vi "seebeck.vi"() -> ()   [LabVIEW 2023]
uses:
  <instrlib>/Keithley 622x LV 2009/Keithley 622x.lvlib
  <instrlib>/Keithley 622x LV 2009/Utility/Typedefs/KE622x -- Instrument Type.ctl
  <vilib>/Analysis/NI_AALBase.lvlib
  <vilib>/Analysis/1siggen.llb/Ramp Pattern by Samples.vi
  Global Variables/MQM Data Transfer All.vi
  <vilib>/Analysis/baseanly.llb/Mean (DBL).vi
  Typedefs/Kxx_Kxy_state_machine_cases.ctl
  Global Variables/Thermometers.vi
  <vilib>/Utility/file.llb/Read Delimited Spreadsheet (DBL).vi
  <vilib>/Instr/_visa.llb/VISA Configure Serial Port (Instr).vi
  <vilib>/Utility/file.llb/Write To Spreadsheet File (string).vi
  Global Variables/KE2182 Voltage.vi
panel:
  in  "Seebeck Voltage Array":dbl[](array[numeric])
  in  "Seebeck coeff data":dbl[](array[numeric])
  in  "T_avg data":dbl[](array[numeric])
  in  "dTxx":dbl
  in  "HTR Power":dbl
  in  "T_avg":dbl
  in  "T_H Array":dbl[](array[numeric])
  in  "T_C Array":dbl[](array[numeric])
  in  "Seebeck Voltage":dbl
  in  "?":enum32{"Setup", "Plotting", "Error Readouts"}(tab)
  in  "DeltaT (fraction of tsp)":dbl=0.05
  in  "Heater Current File (H, T, current)":path
  out "Heater Current \nArray":dbl[](array[numeric])
  out "Ramp Pattern":dbl[](array[numeric])
  in  "Tstart (K)":dbl=3.0
  in  "Tend (K)":dbl=4.0
  in  "Steps":i16=2
  in  "Log (on)\nLin (off) (Temperature setpoints)":bool=TRUE
  in  "Initial Heater Current (A)":dbl=1e-06
  in  "Hstart (Oe)":dbl
  in  "Hend (Oe)":dbl
  in  "Field Steps":i16=1
  in  "Log (on)\nLin (off)  (Field setpoints)":bool
  in  "Test?":bool
  in  "Calibration Only?":bool
  in  "Exchange gas?":bool
  in  "Preset Heater Current Array?":bool
  in  "T Current Source":refnum<visa-resource-name>="6221B"
  in  "HTR Current Source":refnum<visa-resource-name>="CS580-1"
  in  "Thermometer Frequency (Hz)":string="37"
  in  "Initial Thermometer Current (A)":string="1.4142e-7"
  in  "Final Field (Oe)":dbl
  in  "Final Temperature (K)":dbl=1.7
  in  "Filename":path=path "C:/User Data/Luke/Kxx/NaYSe2/NaYSe2_1p7_100K_log_100_9T_8_23_21"
  in  "Heater Only?":bool
  in  "Running avg size":dbl=500.0 format="%#_13g"
  in  "std/mean thresh":dbl=1e-05 format="%#_13g"
  in  "slope/mean thresh":dbl=1e-07 format="%#_13g"
  out "Seebeck Coeff Plot":cluster{dbl[], dbl[]}(graph)
  out "All Data":cluster{dbl[], dbl[]}[](graph)
  in  "Finish":bool
  out "Data Rate (ms)":u32
  in  "Delay (ms)":dbl=300.0
  in  "Quick Data Recording":bool=TRUE
  out "Tsp":dbl
  out "HTR_Current":dbl
  out "Mask":dbl
  out "Seebeck Voltage":dbl
  out "T_H":dbl
  out "T_C1":dbl
  out "I_therm":dbl
  out "T_C2":dbl
  in  "Display Elements":cluster{"X":bool, "Y":bool, "Name":u16}[](array[cluster]) {"Name" items=["Time (ms)", "Temperature (K)", "Field (T)", "LI_1_X", "LI_1_theta", "LI_2_X", "LI_2_theta", "LI_3_X", "LI_3_theta", "DC_V", "DC_I", "mask", "tsp", "I_therm", "T_H", "T_C1", "T_C2", "Fieldsp"]}
  in  "X-Axis":u16(ring) items=["Linear", "Reciprocal", "Log10"]
  in  "Y-Axis":u16(ring) items=["Linear", "Reciprocal", "Log10"]
  out "Fieldsp":dbl
  out "Global Stop":bool
  out "Thermometers":cluster{"T_H":dbl, "T_C1":dbl, "T_C2":dbl}
  out "QD error out":errorcluster
  out "KE6221 error out":errorcluster
  # "TURN ON HIGH VACUUM!"
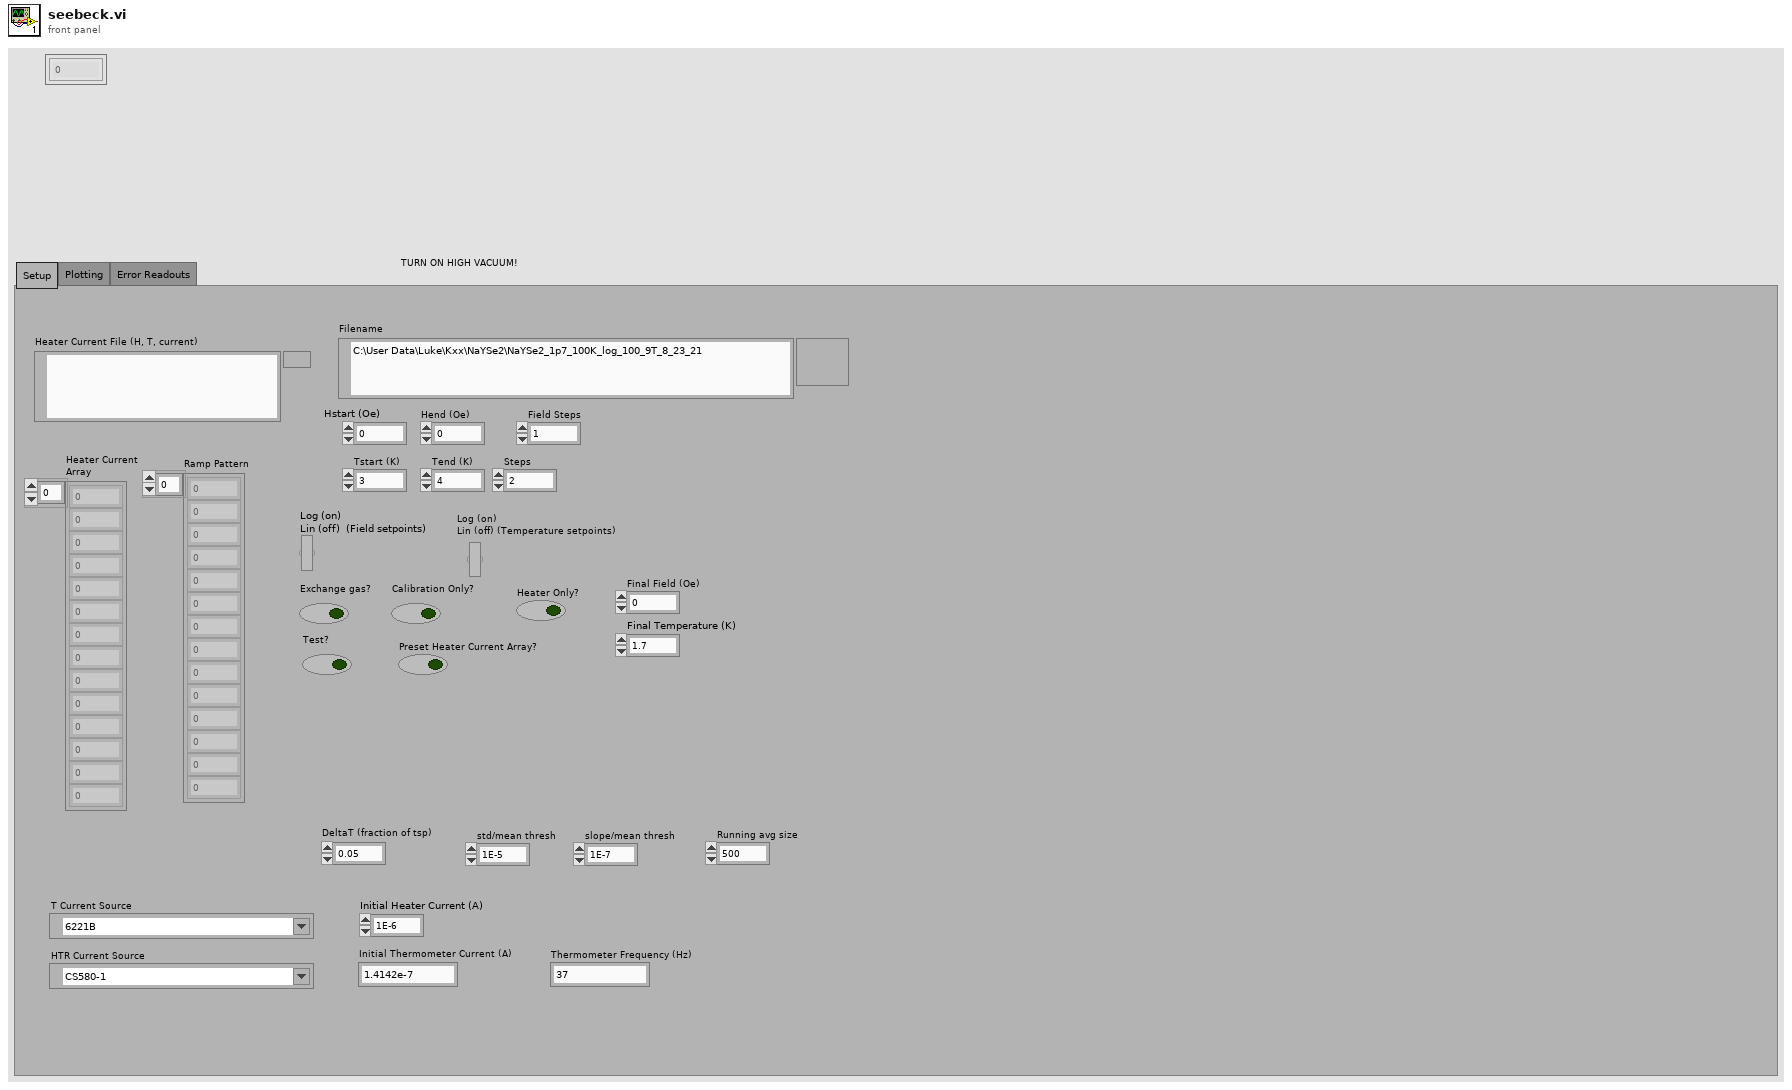
[diagram p1: front panel]
types:
  T1 = typedef "Keithley 622x.lvlib/KE622x -- Instrument Type.ctl" = enum16{"KE6220", "KE6221"}
  T2 = typedef "Kxx_Kxy_state_machine_cases.ctl" = enum16{"Initialize", "Wait to Stabilize (no heat)", "Measure (no heat)", "Turn on Heater, stabilize", "Measure (heat)", "Turn off Heater", "Assign Heater Current", "Plot", "End"}
  T3 = cluster{"T_avg data":dbl[], "Seebeck coeff data":dbl[]}
  T4 = cluster{"T_avg":dbl, "dTxx":dbl, "HTR Power":dbl, "Seebeck Voltage":dbl, "T_H Array":dbl[], "T_C Array":dbl[], "Seebeck Voltage Array":dbl[], "error out":errorcluster}
  T5 = typedef "ZI_Frontpanel_All.ctl" = cluster{"Lockin 1 Demod 0":cluster{"R(V)":dbl, "Theta (deg)":dbl, "Timestamp (ms)":u32, "X(V)":dbl, "Y(V)":dbl, "frequency (Hz)":dbl, "output voltage (V)":dbl}, "Lockin 2 Demod 0":cluster{"R(V)":dbl, "Theta (deg)":dbl, "Timestamp (ms)":u32, "X(V)":dbl, "Y(V)":dbl, "frequency (Hz)":dbl, "output voltage (V)":dbl}, "Lockin 3 Demod 0":cluster{"R(V)":dbl, "Theta (deg)":dbl, "Timestamp (ms)":u32, "X(V)":dbl, "Y(V)":dbl, "frequency (Hz)":dbl, "output voltage (V)":dbl}, "Lockin 4 Demod 0":cluster{"R(V)":dbl, "Theta (deg)":dbl, "Timestamp (ms)":u32, "X(V)":dbl, "Y(V)":dbl, "frequency (Hz)":dbl, "output voltage (V)":dbl}, "LI1 active":bool, "LI2 active":bool, "LI3 active":bool, "LI4 active":bool}
  T6 = typedef "PPMS_Status.ctl" = cluster{"Field":cluster{"Field (T)":dbl, "Field stable":bool, "Timestamp (ms)":u32}, "Temperature":cluster{"Temperature (K)":dbl, "Temperature stable":bool, "Timestamp (ms)":u32}}
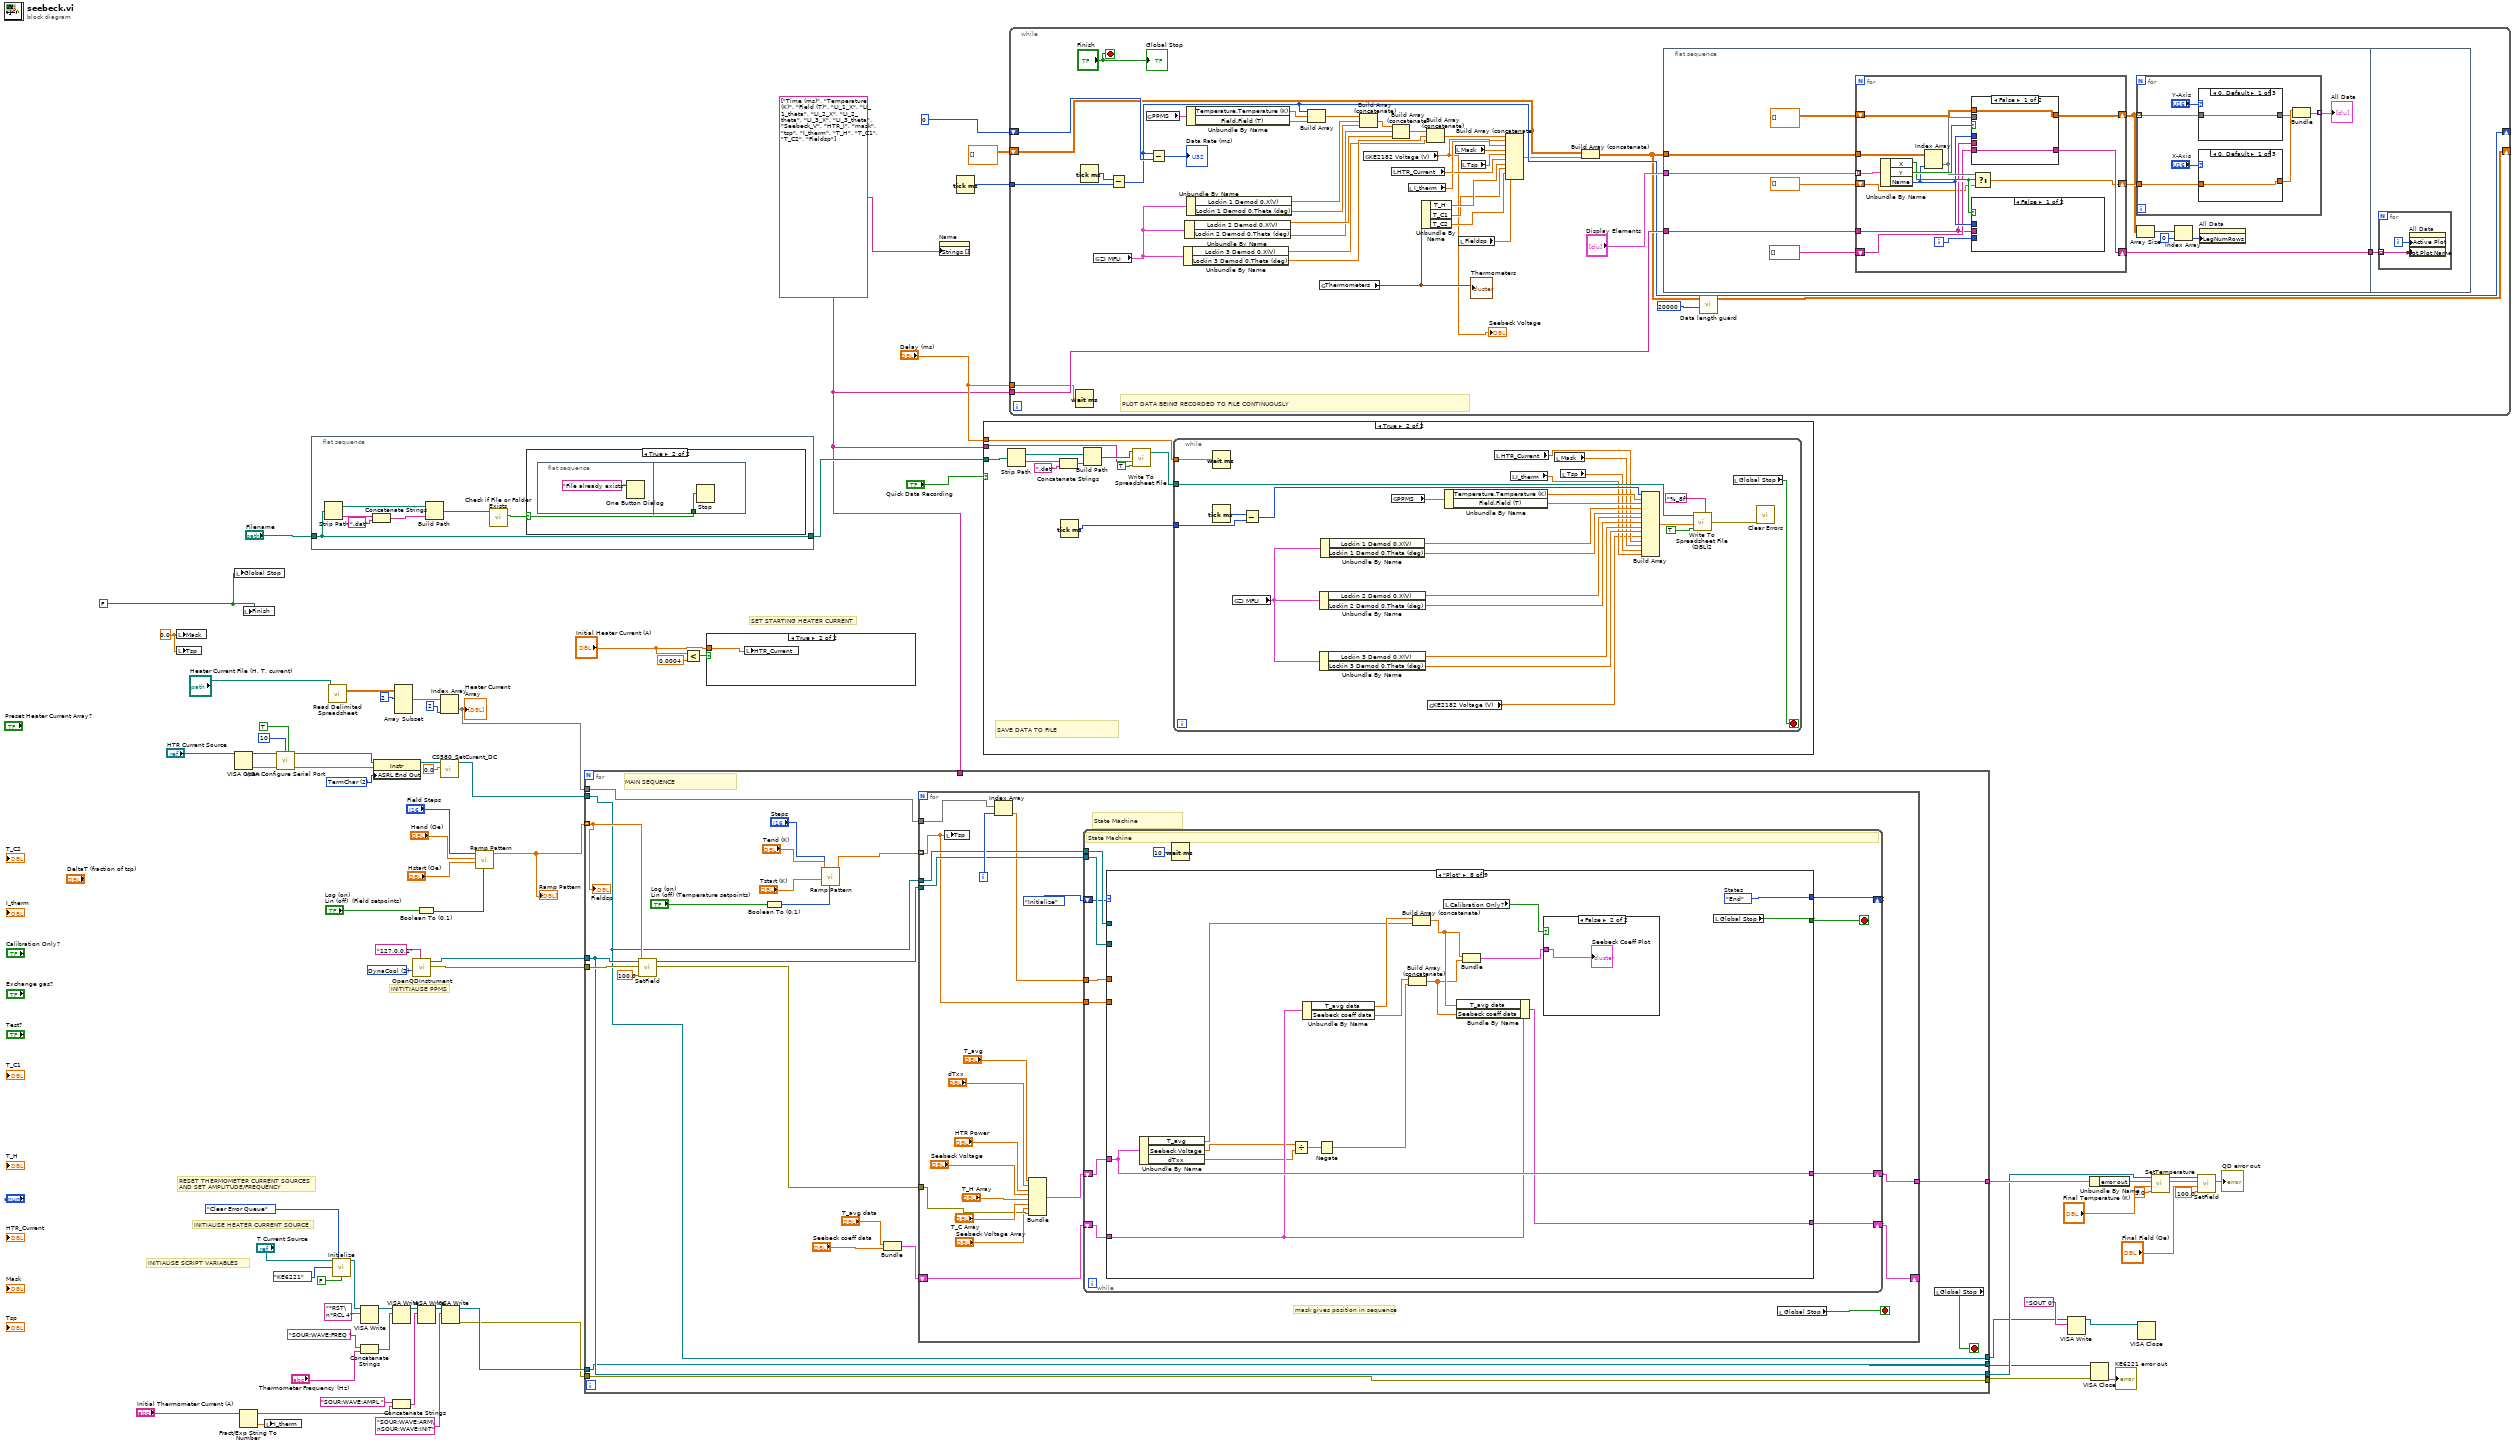
[diagram p0: block diagram]
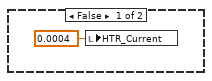
[diagram p2: hidden frame]
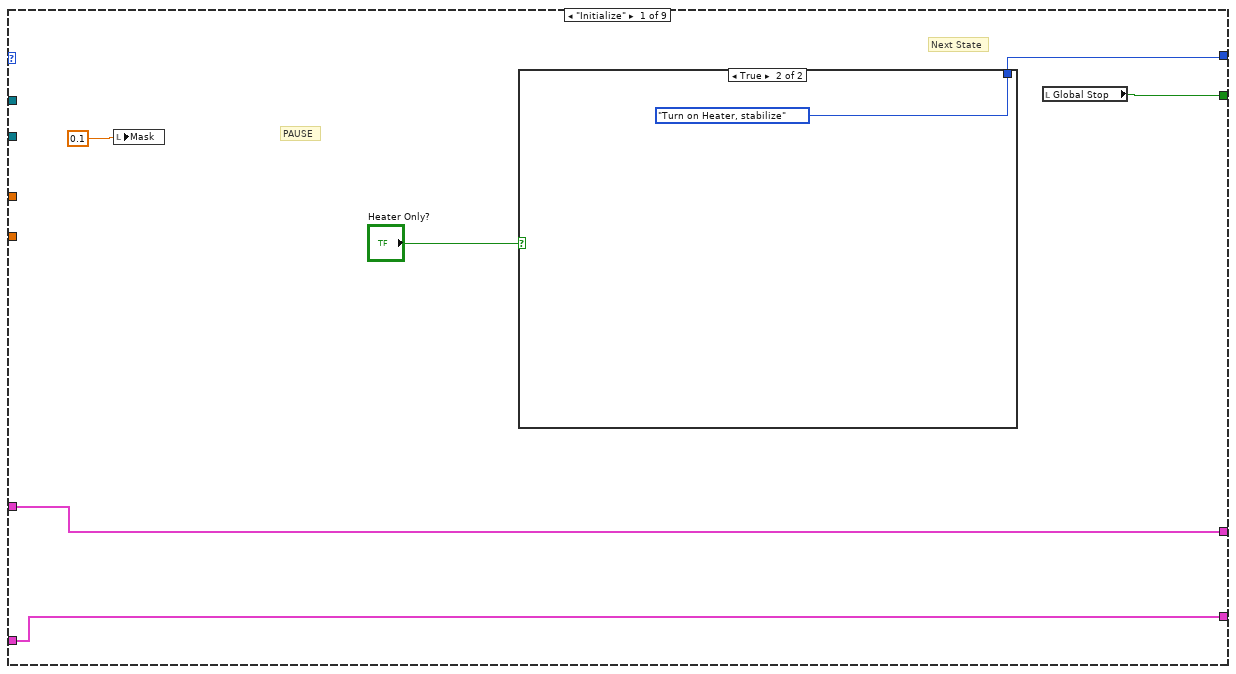
[diagram p4: hidden frame]
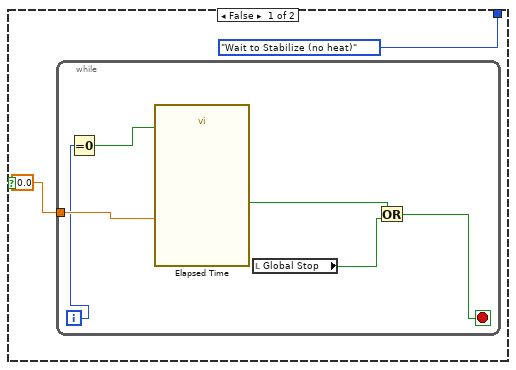
[diagram p5: hidden frame]
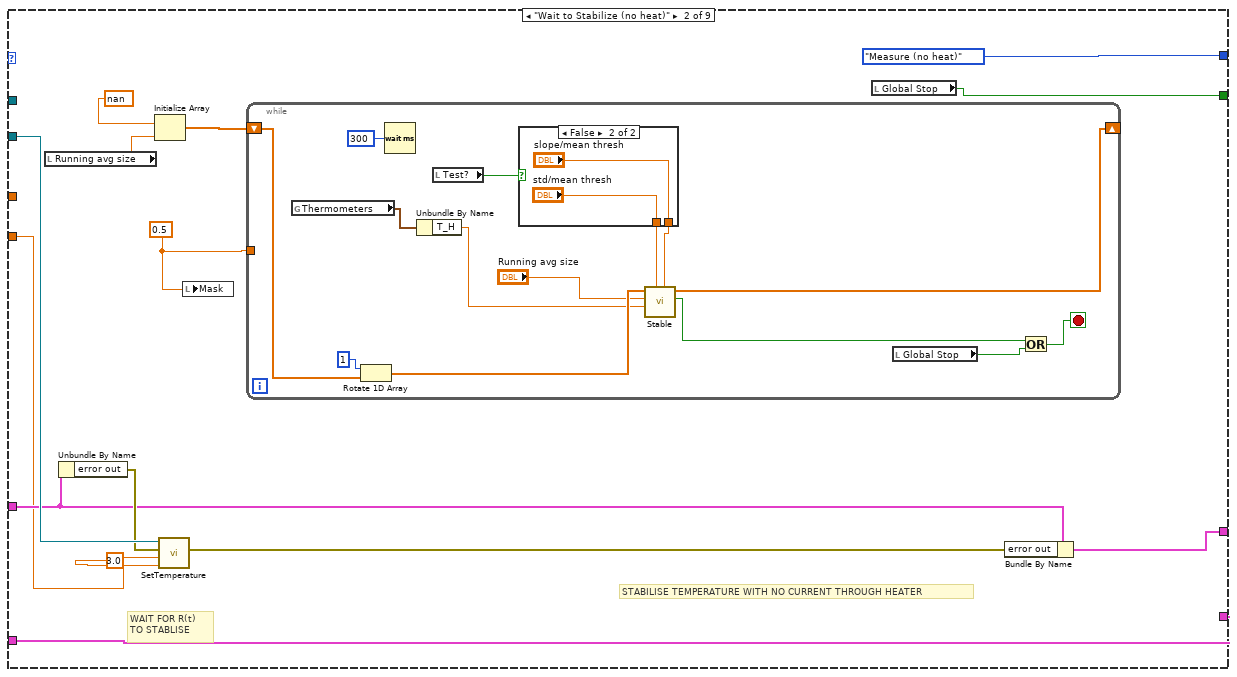
[diagram p6: hidden frame]
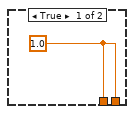
[diagram p7: hidden frame]
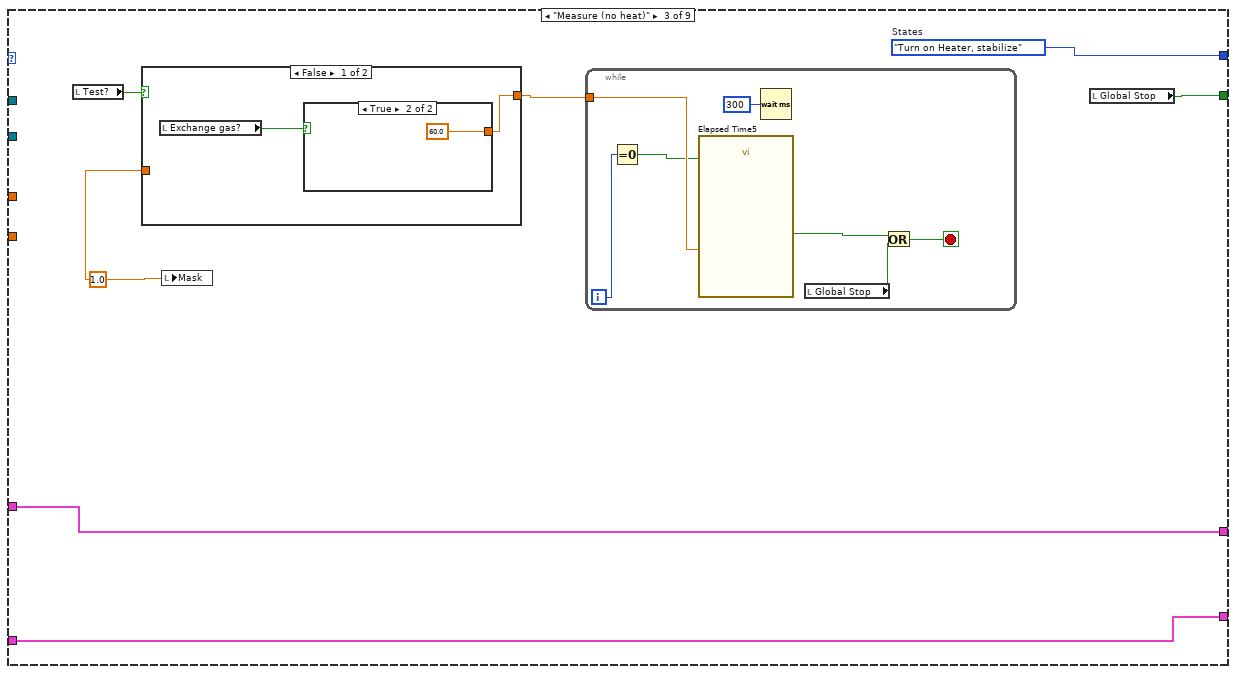
[diagram p8: hidden frame]
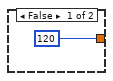
[diagram p9: hidden frame]
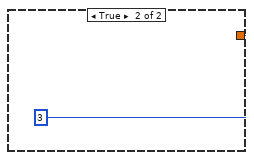
[diagram p10: hidden frame]
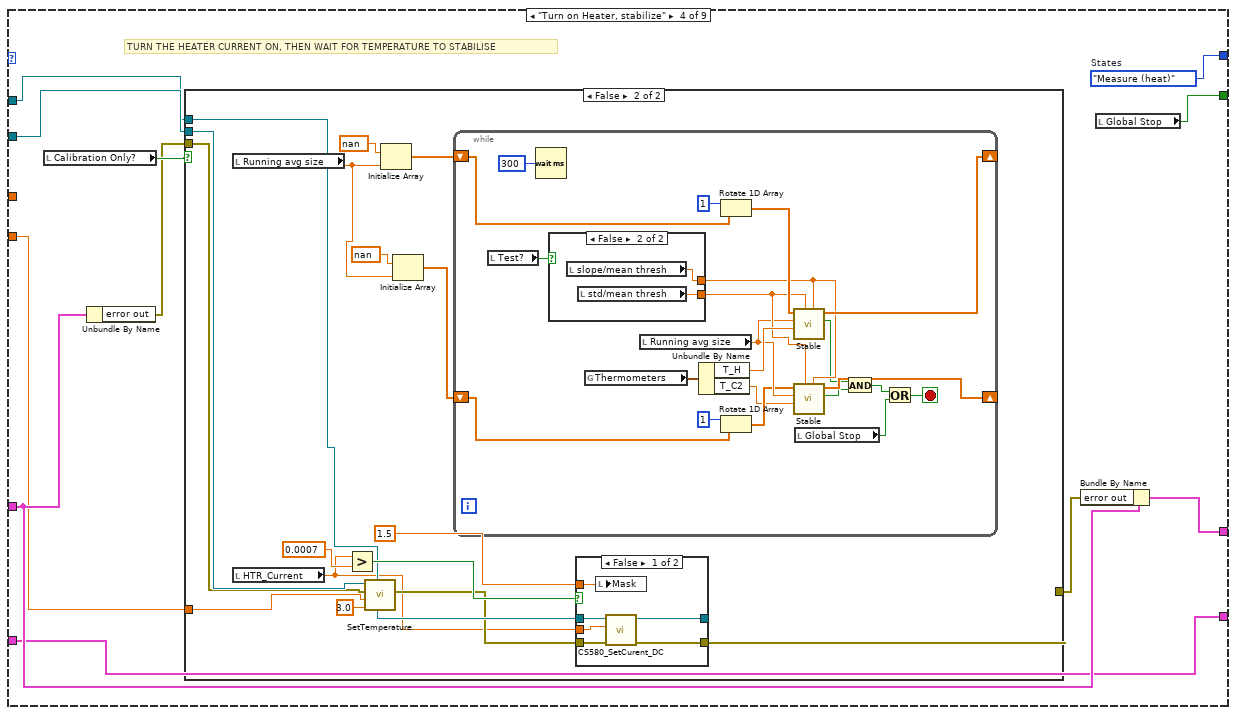
[diagram p11: hidden frame]
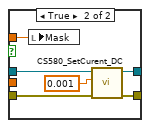
[diagram p13: hidden frame]
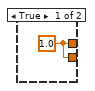
[diagram p14: hidden frame]
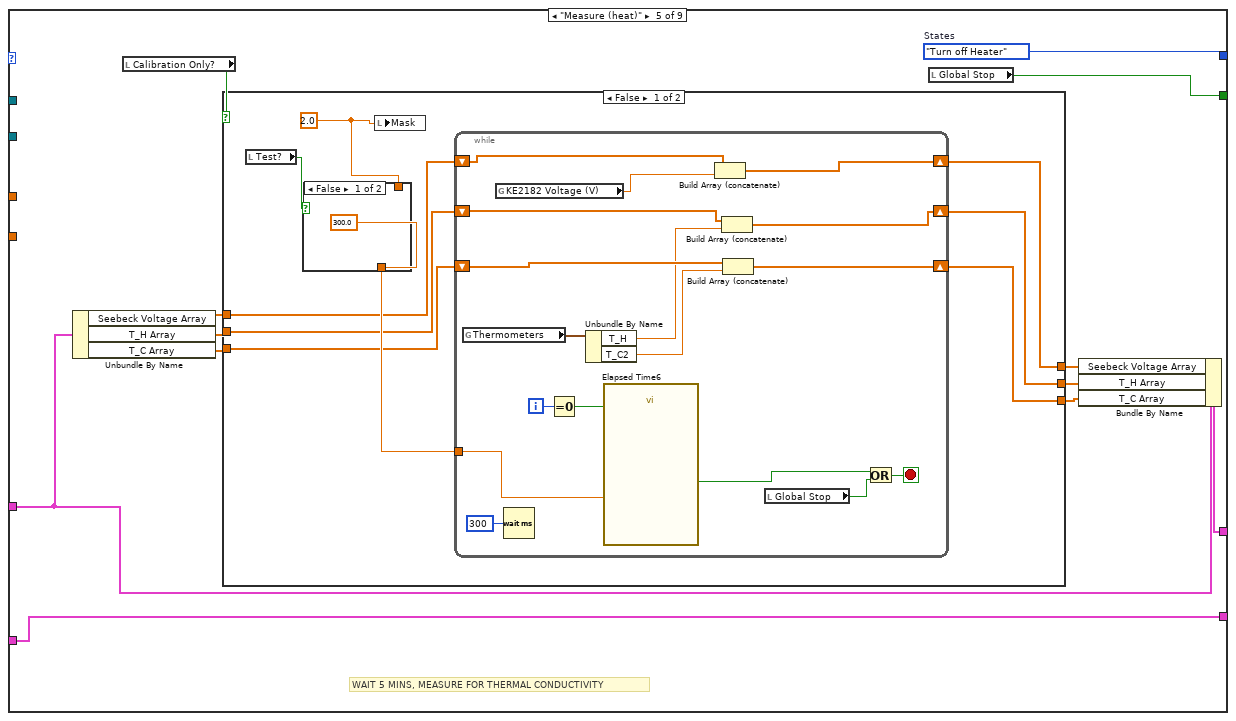
[diagram p15: hidden frame]
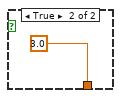
[diagram p16: hidden frame]
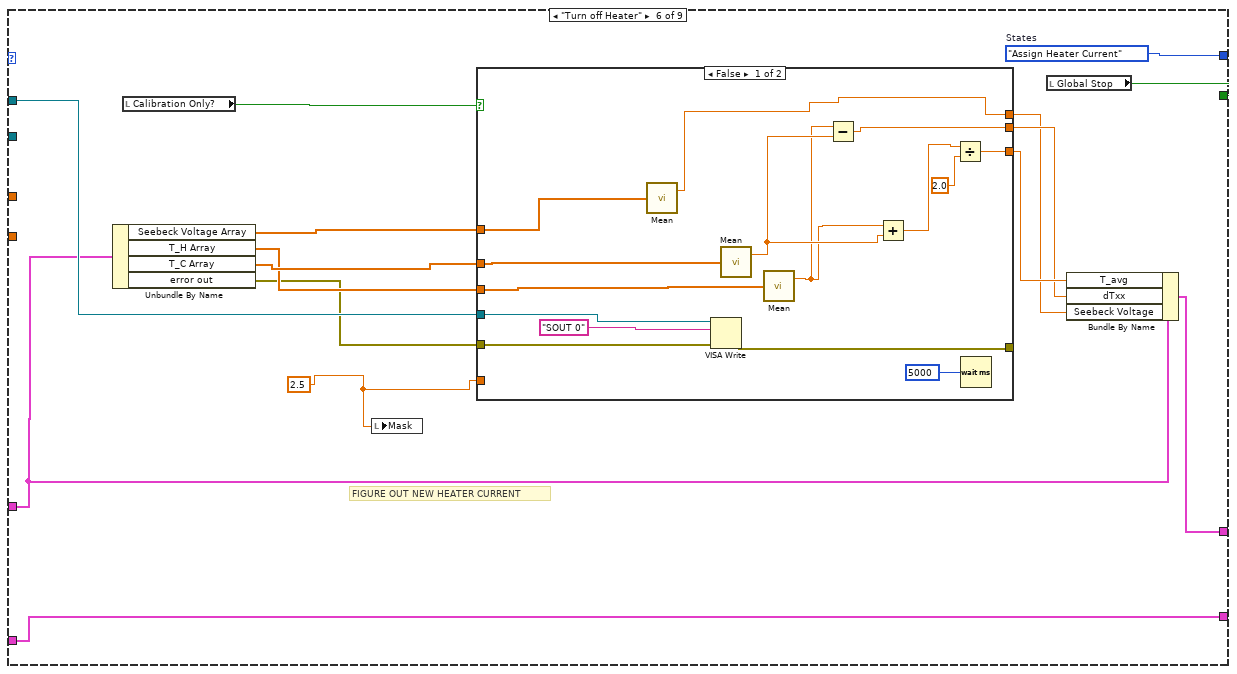
[diagram p18: hidden frame]
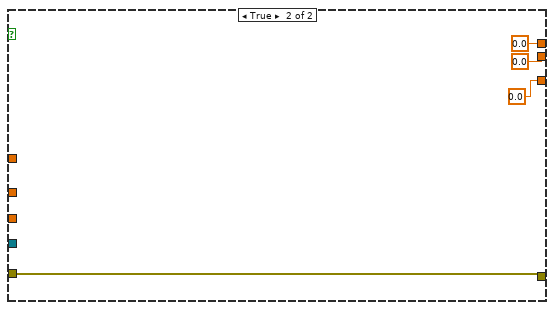
[diagram p19: hidden frame]
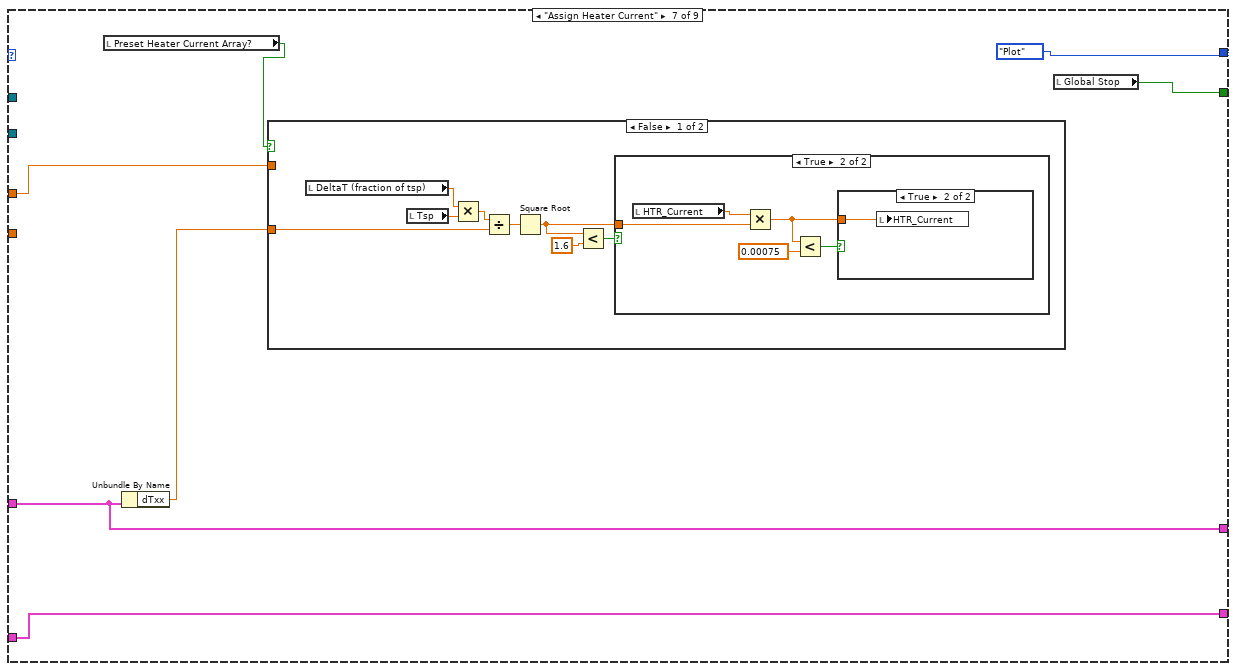
[diagram p20: hidden frame]
diagram:
  w6 = FALSE ("Calibration confirmed")
  w5 = string[] ["Time (ms)", "Temperature (K)", "Field (T)", "LI_1_X", "LI_1_theta", "LI_2_X", "LI_2_theta", "LI_3_X", "LI_3_theta", "Seebeck_V", "HTR_I", "mask", "tsp", "I_therm", "T_H", "T_C1", "T_C2", "Fieldsp"] ("element")
  w51 = u16 2 items=["None", "Last Bit", "TermChar", "Break"] ("Serial Settings:End Mode for Writes")
  w69 = 0.0 ("Mask")
  w71 = 2 items=["PPMS", "VersaLab", "DynaCool", "SVSM"] ("Instrument Type")
  # "SET STARTING HEATER CURRENT"
  # "INITIALISE HEATER CURRENT SOURCE"
  # "RESET THERMOMETER CURRENT SOURCES\nAND SET AMPLITUDE/FREQUENCY"
  # "INITITIALISE PPMS"
  # "INITIALISE SCRIPT VARIABLES"
  n1 = local write "Mask"(w69) -> ()
  n2 = local write "Tsp"(w69) -> ()
  n3 = VISA Open(VISA resource name="HTR Current Source") -> (VISA resource name=w47:refnum<visa-resource-name>, error out=w48:errorcluster)  [unwired: 4 in]
  n4 = local write "Global Stop"(w6) -> ()
  n5 = Fract/Exp String To Number(string="Initial Thermometer Current (A)") -> (number=w59:dbl)  [unwired: 3 in, 1 out]
  n6 = local write "Finish"(w6) -> ()
  n7 = local write "I_therm"(w59) -> ()
  n8 = call-poly "VISA Configure Serial Port"("VISA resource name"=w47, "termination char\n(0xA = '\\n' = LF)"=u8 10 ("termination char\n(0xA = '\\n' = LF)"), "Enable Termination\nChar (T)"=TRUE ("Enable Termination\nChar (T)"), "error in (no error)"=w48) -> ("VISA resource name out"=w49:refnum<visa-resource-name>, "error out"=w50:errorcluster)  [unwired: 10 in]
  n9 = flat-sequence {
    tunnel: "Filename" -> [w78]
    tunnel: [w78] -> w22
    frame #0 {
      n10 = Strip Path(path=w78) -> (stripped path=w82:path, name=w79:string)
      n11 = Concatenate Strings(w79, ".dat") -> (w81:string)
      n12 = Build Path(base path=w82, name or relative path=w81) -> (appended path=w77:path)
      n13 = call <vilib>:"Check if File or Folder Exists.vi"("path"=w77) -> ("file or folder exists?"=w76:bool)  [unwired: 8 in, 2 out]
      n14 = case shown="True" w76 {
        selector: w76 -> [_ w83]
        frame False {
        }
        frame True {
          n15 = flat-sequence {
            tunnel: w83 -> [w85]
            frame #0 {
              n16 = One Button Dialog(message="File already exists") -> ()  [unwired: 1 in, 1 out]
            }
            frame #1 {
              n17 = Stop(stop? (T)=w85) -> ()
            }
          }
        }
      }
    }
  }
  n18 = call-poly <vilib>:"Read Delimited Spreadsheet.vi"("file path (dialog if empty)"="Heater Current File (H, T, current)") -> ("all rows"=w42:dbl[][])  [unwired: 9 in, 5 out]
  n19 = call <instrlib>:"Initialize.vi"("VISA resource name"="T Current Source", "Error Queue Option"=enum16{"Clear Error Queue", "Error Query"}."Clear Error Queue", "Instrument Type"=KE622x_--_Instrument_Type."KE6221", "Reset? (T)"=FALSE) -> ("VISA resource name out"=w67:refnum<visa-resource-name>)  [unwired: 10 in, 1 out]
  n20 = VISA Write(VISA resource name=w67, write buffer="*RST\n*RCL 4") -> (VISA resource name out=w61:refnum<visa-resource-name>)  [unwired: 1 in, 2 out]
  n21 = Concatenate Strings("SOUR:WAVE:FREQ " ("string"), "Thermometer Frequency (Hz)") -> (w66:string)
  n22 = property class="Instr"(reference=w49, error in=w50, "ASRL End Out"=w51) -> (reference out=w45:refnum<visa-resource-name>)  [unwired: 1 out]
  n23 = VISA Write(VISA resource name=w61, write buffer=w66) -> (VISA resource name out=w60:refnum<visa-resource-name>)  [unwired: 1 in, 2 out]
  n24 = Concatenate Strings("SOUR:WAVE:AMPL " ("string"), "Initial Thermometer Current (A)") -> (w63:string)
  n25 = Array Subset(array=w42, index (row)=2 ("index")) -> (w40:dbl[][])  [unwired: 3 in]
  n26 = call <instrlib>:"OpenQDInstrument.vi"("IP Address"="127.0.0.1", "Instrument Type"=w71) -> ("error out"=w21:errorcluster, "Instrument Ref"=w19:refnum<k24>)  [unwired: 6 in]
  n27 = VISA Write(VISA resource name=w60, write buffer=w63) -> (VISA resource name out=w37:refnum<visa-resource-name>)  [unwired: 1 in, 2 out]
  n28 = Boolean To (0,1)(Boolean="Log (on)\nLin (off)  (Field setpoints)") -> (0, 1=w54:i16)
  n29 = Index Array(array=w40, index (col)=2 ("disabled index (col)")) -> (element=w35:dbl[])  [unwired: 1 in]
  "Heater Current \nArray" <- w35
  n30 = call "CS580_SetCurent_DC.vi"("Current (A)"=0.0, "VISA Refnum in"=w45) -> ("VISA resource name out"=w20:refnum<visa-resource-name>)  [unwired: 8 in, 1 out]
  n31 = VISA Write(VISA resource name=w37, write buffer="SOUR:WAVE:ARM\nSOUR:WAVE:INIT") -> (VISA resource name out=w13:refnum<visa-resource-name>, error out=w9:errorcluster)  [unwired: 1 in, 1 out]
  n32 = call-poly <vilib>:"Ramp Pattern.vi"("type"=w54, "start"="Hstart (Oe)", "end"="Hend (Oe)", "samples"="Field Steps") -> ("Ramp Pattern"=w36:dbl[])  [unwired: 6 in, 1 out]
  "Ramp Pattern" <- w36
  n33 = for {
    tunnel: w36 -> [w106] mode=indexing
    tunnel: w19 -> [w90]
    tunnel: w21 -> [w104]
    tunnel: w35 -> [w97]
    tunnel: w20 -> [w86]
    tunnel: [w91] -> w15
    tunnel: w13 -> [w89]
    tunnel: [w90] -> w12
    tunnel: [w89] -> w11
    tunnel: w9 -> [w88]
    tunnel: [w88] -> w8
    tunnel: [w86] -> w3
    tunnel: w5 -> [_]
    stop <- w87 stop-if-true
    # "MAIN SEQUENCE"
    n34 = call <instrlib>:"SetField.vi"("Rate"=100.0, "Field"=w106, "error in (no error)"=w104, "Instrument Ref In"=w90) -> ("error out"=w96:errorcluster, "Instrument Ref Out"=w95:refnum<k24>)  [unwired: 3 in, 1 out]
    n35 = Boolean To (0,1)(Boolean="Log (on)\nLin (off) (Temperature setpoints)") -> (0, 1=w101:i16)
    n36 = call-poly <vilib>:"Ramp Pattern.vi"("type"=w101, "start"="Tstart (K)", "end"="Tend (K)", "samples"="Steps") -> ("Ramp Pattern"=w103:dbl[])  [unwired: 6 in, 1 out]
    n37 = Bundle("T_avg data"="T_avg data", "Seebeck coeff data"="Seebeck coeff data") -> (w92:T3)  [unwired: 1 in]
    n38 = for {
      tunnel: w103 -> [w115] mode=indexing
      tunnel: w97 -> [w126]
      tunnel: w96 -> [w108]
      tunnel: w86 -> [w124]
      tunnel: w95 -> [w123]
      shift-right: [w114] -> _
      shift-left: w92 -> [w113]
      tunnel: [w117] -> w91
      i -> [w125]
      stop <- w116 stop-if-true
      # "State Machine"
      # "mask gives position in sequence"
      n39 = local write "Tsp"(w115) -> ()
      n40 = Index Array(array=w126, index=w125) -> (element=w118:dbl)
      n41 = Bundle("T_avg"="T_avg", "dTxx"="dTxx", "HTR Power"="HTR Power", "Seebeck Voltage"="Seebeck Voltage", "T_H Array"="T_H Array", "T_C Array"="T_C Array", "Seebeck Voltage Array"="Seebeck Voltage Array", "error out"=w108) -> (w119:T4)  [unwired: 1 in]
      n42 = while {
        shift-right: [w138] -> _
        shift-left: Kxx_Kxy_state_machine_cases."Initialize" -> [w127]
        tunnel: w124 -> [w136]
        tunnel: w123 -> [w132]
        shift-right: [w135] -> w117
        shift-left: w119 -> [w134]
        tunnel: w118 -> [w133]
        tunnel: w115 -> [w130]
        shift-right: [w129] -> w114
        shift-left: w113 -> [w128]
        stop <- w131 stop-if-true
        # "State Machine"
        n43 = case shown="\"Plot\"" w127 {
          selector: w127 -> [_ _ _ _ _ _ _ _ w391]
          tunnel: w132 -> [_ w163 _ w213 _ _ _ _ _]
          tunnel: [w143 Kxx_Kxy_state_machine_cases."Measure (no heat)" w189 w211 w278 w323 Kxx_Kxy_state_machine_cases."Plot" w384 w391] -> w138
          tunnel: w136 -> [_ _ _ w212 _ w324 _ _ _]
          tunnel: [w142 w159 w188 w207 w272 w318 w349 w383 w390] -> w135
          tunnel: w134 -> [w142 w160 w188 w209 w271 w319 w349 w383 w390]
          tunnel: w128 -> [w141 w158 w187 w206 w270 w317 w348 w380 w389]
          tunnel: [w141 w158 w187 w206 w270 w317 w348 w379 w389] -> w129
          tunnel: w133 -> [_ _ _ _ _ _ w347 _ _]
          tunnel: [w140 w157 w186 w205 w269 w316 w346 w378 TRUE] -> w131
          tunnel: w130 -> [_ w156 _ w204 _ _ _ _ _]
          frame "Initialize" {
            # "Next State"
            # "PAUSE"
            n44 = local write "Mask"(0.1 ("Mask")) -> ()
            n45 = case shown="True" "Heater Only?" {
              tunnel: [Kxx_Kxy_state_machine_cases."Wait to Stabilize (no heat)" Kxx_Kxy_state_machine_cases."Turn on Heater, stabilize"] -> w143
              frame False {
                n46 = while {
                  tunnel: 10.0 ("Time Target (s)") -> [w152]
                  i -> [w148]
                  stop <- w149 stop-if-true
                  n47 = Equal To 0?(x=w148) -> (x = 0?=w147:bool)
                  n48 = call "Elapsed Time"("Time Target (s)"=w152, "Reset"=w147) -> ("Time has Elapsed"=w151:bool)  [unwired: 10 in, 7 out]
                  n49 = local read "Global Stop"() -> (w150:bool)
                  n50 = Or(x=w151, y=w150) -> (x .or. y?=w149:bool)
                }
              }
              frame True {
              }
            }
            n51 = local read "Global Stop"() -> (w140:bool)
          }
          frame "Wait to Stabilize (no heat)" {
            w154 = 0.5 ("Mask")
            # "STABILISE TEMPERATURE WITH NO CURRENT THROUGH HEATER"
            # "WAIT FOR R(t)\nTO STABLISE"
            n52 = local read "Running avg size"() -> (w165:dbl)
            n53 = Unbundle By Name(w160) -> ("error out"=w161:errorcluster)
            n54 = Initialize Array(nan ("Element"), w165) -> (w167:dbl[])
            n55 = call <instrlib>:"SetTemperature.vi"("Rate"=3.0, "Temperature"=w156, "error in (no error)"=w161, "Instrument Ref In"=w163) -> ("error out"=w155:errorcluster)  [unwired: 3 in, 2 out]
            n56 = local write "Mask"(w154) -> ()
            n57 = while {
              shift-right: [w170] -> _
              shift-left: w167 -> [w180]
              tunnel: w154 -> [_]
              stop <- w176 stop-if-true
              n58 = global read "Thermometers.vi" "Thermometers"() -> (w175:cluster{"T_H":dbl, "T_C1":dbl, "T_C2":dbl})
              n59 = Rotate 1D Array(1:w180, 2:1 ("n")) -> (0:w174:dbl[])
              n60 = Wait (ms)(milliseconds to wait=u32 300) -> ()  [unwired: 1 out]
              n61 = Unbundle By Name(w175) -> ("T_H"=w172:dbl)
              n62 = local read "Test?"() -> (w178:bool)
              n63 = case shown="False" w178 {
                tunnel: [w182 "slope/mean thresh"] -> w171
                tunnel: [w182 "std/mean thresh"] -> w168
                frame True {
                  w182 = 1.0 ("y")
                }
                frame False {
                }
              }
              n64 = call "Stable.vi"("slope/mean thresh"=w171, "std/mean thresh"=w168, "New data point"=w172, "Number of points"="Running avg size", "Array in"=w174) -> ("Stable?"=w169:bool, "Array out"=w170:dbl[])  [unwired: 5 in]
              n65 = local read "Global Stop"() -> (w177:bool)
              n66 = Or(x=w169, y=w177) -> (x .or. y?=w176:bool)
            }
            n67 = local read "Global Stop"() -> (w157:bool)
            n68 = Bundle By Name(cluster=w160, "error out"=w155) -> (w159:T4)
          }
          frame "Measure (no heat)" {
            w189 = Kxx_Kxy_state_machine_cases."Turn on Heater, stabilize"  # States
            w185 = 1.0 ("Mask")
            n69 = local read "Test?"() -> (w191:bool)
            n70 = case shown="False" w191 {
              tunnel: [w192 u32 3 ("milliseconds to wait")] -> w190
              tunnel: w185 -> [_ _]
              frame False {
                n71 = local read "Exchange gas?"() -> (w193:bool)
                n72 = case shown="True" w193 {
                  tunnel: [120 60.0 ("Time to Wait (s)")] -> w192
                  frame False {
                  }
                  frame True {
                  }
                }
              }
              frame True {
              }
            }
            n73 = local write "Mask"(w185) -> ()
            n74 = while {
              tunnel: w190 -> [w201]
              i -> [w198]
              stop <- w200 stop-if-true
              n75 = Equal To 0?(x=w198) -> (x = 0?=w197:bool)
              n76 = call "Elapsed Time5"("Time Target (s)"=w201, "Reset"=w197) -> ("Time has Elapsed"=w199:bool)  [unwired: 10 in, 7 out]
              n77 = Wait (ms)(milliseconds to wait=u32 300) -> ()  [unwired: 1 out]
              n78 = local read "Global Stop"() -> (w203:bool)
              n79 = Or(x=w199, y=w203) -> (x .or. y?=w200:bool)
            }
            n80 = local read "Global Stop"() -> (w186:bool)
          }
          frame "Turn on Heater, stabilize" {
            w211 = Kxx_Kxy_state_machine_cases."Measure (heat)"  # States
            # "TURN THE HEATER CURRENT ON, THEN WAIT FOR TEMPERATURE TO STABILISE"
            n81 = local read "Calibration Only?"() -> (w214:bool)
            n82 = Unbundle By Name(w209) -> ("error out"=w210:errorcluster)
            n83 = case shown="False" w214 {
              tunnel: w213 -> [_ w231]
              tunnel: w210 -> [w215 w224]
              tunnel: [w215 w225] -> w208
              tunnel: w212 -> [_ w226]
              tunnel: w204 -> [_ w221]
              frame True {
              }
              frame False {
                n84 = local read "Running avg size"() -> (w216:dbl)
                n85 = local read "HTR_Current"() -> (w219:dbl)
                n86 = Greater?(x=w219, y=0.0007) -> (0:w227:bool)
                n87 = call <instrlib>:"SetTemperature.vi"("Rate"=3.0, "Temperature"=w221, "error in (no error)"=w224, "Instrument Ref In"=w231) -> ("error out"=w223:errorcluster)  [unwired: 3 in, 2 out]
                n88 = Initialize Array(nan ("Element"), w216) -> (w230:dbl[])
                n89 = Initialize Array(nan ("Element"), w216) -> (w217:dbl[])
                n90 = while {
                  shift-right: [w261] -> _
                  shift-left: w230 -> [w263]
                  shift-right: [w248] -> _
                  shift-left: w217 -> [w251]
                  stop <- w259 stop-if-true
                  n91 = local read "Test?"() -> (w260:bool)
                  n92 = Wait (ms)(milliseconds to wait=u32 300) -> ()  [unwired: 1 out]
                  n93 = case shown="False" w260 {
                    tunnel: [w265 w267] -> w254
                    tunnel: [w265 w266] -> w253
                    frame True {
                      w265 = 1.0 ("y")
                    }
                    frame False {
                      n94 = local read "slope/mean thresh"() -> (w267:dbl)
                      n95 = local read "std/mean thresh"() -> (w266:dbl)
                    }
                  }
                  n96 = global read "Thermometers.vi" "Thermometers"() -> (w257:cluster{"T_H":dbl, "T_C1":dbl, "T_C2":dbl})
                  n97 = local read "Running avg size"() -> (w252:dbl)
                  n98 = Unbundle By Name(w257) -> ("T_H"=w255:dbl, "T_C2"=w244:dbl)
                  n99 = Rotate 1D Array(1:w263, 2:1 ("n")) -> (0:w256:dbl[])
                  n100 = Rotate 1D Array(1:w251, 2:1 ("n")) -> (0:w249:dbl[])
                  n101 = call "Stable.vi"("slope/mean thresh"=w254, "std/mean thresh"=w253, "New data point"=w255, "Number of points"=w252, "Array in"=w256) -> ("Stable?"=w247:bool, "Array out"=w261:dbl[])  [unwired: 5 in]
                  n102 = call "Stable.vi"("slope/mean thresh"=w254, "std/mean thresh"=w253, "New data point"=w244, "Number of points"=w252, "Array in"=w249) -> ("Stable?"=w246:bool, "Array out"=w248:dbl[])  [unwired: 5 in]
                  n103 = local read "Global Stop"() -> (w258:bool)
                  n104 = And(x=w247, y=w246) -> (x .and. y?=w245:bool)
                  n105 = Or(x=w245, y=w258) -> (x .or. y?=w259:bool)
                }
                n106 = case shown="False" w227 {
                  tunnel: w223 -> [w235 w243]
                  tunnel: w226 -> [w236 w242]
                  tunnel: [w233 w241] -> w225
                  tunnel: [w234 w240] -> _
                  tunnel: w219 -> [w237 _]
                  tunnel: 1.5 ("Mask") -> [w232 w238]
                  frame False {
                    n107 = local write "Mask"(w232) -> ()
                    n108 = call "CS580_SetCurent_DC.vi"("error in"=w235, "Current (A)"=w237, "VISA Refnum in"=w236) -> ("error out"=w233:errorcluster, "VISA resource name out"=w234:refnum<visa-resource-name>)  [unwired: 7 in]
                  }
                  frame True {
                    n109 = local write "Mask"(w238) -> ()
                    n110 = call "CS580_SetCurent_DC.vi"("error in"=w243, "Current (A)"=0.001, "VISA Refnum in"=w242) -> ("error out"=w241:errorcluster, "VISA resource name out"=w240:refnum<visa-resource-name>)  [unwired: 7 in]
                  }
                }
              }
            }
            n111 = Bundle By Name(cluster=w209, "error out"=w208) -> (w207:T4)
            n112 = local read "Global Stop"() -> (w205:bool)
          }
          frame "Measure (heat)" {
            w278 = Kxx_Kxy_state_machine_cases."Turn off Heater"  # States
            # "WAIT 5 MINS, MEASURE FOR THERMAL CONDUCTIVITY"
            n113 = Unbundle By Name(w271) -> ("Seebeck Voltage Array"=w277:dbl[], "T_H Array"=w276:dbl[], "T_C Array"=w275:dbl[])
            n114 = local read "Calibration Only?"() -> (w279:bool)
            n115 = case shown="False" w279 {
              tunnel: w277 -> [w286 w310]
              tunnel: w276 -> [w283 w309]
              tunnel: w275 -> [w282 w308]
              tunnel: [w285 w310] -> w268
              tunnel: [w281 w309] -> w274
              tunnel: [w280 w308] -> w273
              frame False {
                w284 = 2.0 ("Mask")
                n116 = local read "Test?"() -> (w288:bool)
                n117 = case shown="False" w288 {
                  tunnel: [300.0 3.0] -> w287
                  tunnel: w284 -> [_ _]
                  frame False {
                  }
                  frame True {
                  }
                }
                n118 = local write "Mask"(w284) -> ()
                n119 = while {
                  shift-right: [w306] -> w281
                  shift-left: w283 -> [w307]
                  shift-right: [w304] -> w285
                  shift-left: w286 -> [w305]
                  shift-right: [w299] -> w280
                  shift-left: w282 -> [w300]
                  tunnel: w287 -> [w295]
                  i -> [w302]
                  stop <- w296 stop-if-true
                  n120 = global read "Thermometers.vi" "Thermometers"() -> (w294:cluster{"T_H":dbl, "T_C1":dbl, "T_C2":dbl})
                  n121 = global read "KE2182 Voltage.vi" "KE2182 Voltage (V)"() -> (w291:dbl)
                  n122 = Wait (ms)(milliseconds to wait=u32 300) -> ()  [unwired: 1 out]
                  n123 = Equal To 0?(x=w302) -> (x = 0?=w301:bool)
                  n124 = Unbundle By Name(w294) -> ("T_H"=w293:dbl, "T_C2"=w292:dbl)
                  n125 = call "Elapsed Time6"("Time Target (s)"=w295, "Reset"=w301) -> ("Time has Elapsed"=w298:bool)  [unwired: 10 in, 7 out]
                  n126 = Build Array (concatenate)(w305, w291) -> (w304:dbl[])
                  n127 = Build Array (concatenate)(w307, w293) -> (w306:dbl[])
                  n128 = Build Array (concatenate)(w300, w292) -> (w299:dbl[])
                  n129 = local read "Global Stop"() -> (w297:bool)
                  n130 = Or(x=w298, y=w297) -> (x .or. y?=w296:bool)
                }
              }
              frame True {
              }
            }
            n131 = local read "Global Stop"() -> (w269:bool)
            n132 = Bundle By Name(cluster=w271, "Seebeck Voltage Array"=w268, "T_H Array"=w274, "T_C Array"=w273) -> (w272:T4)
          }
          frame "Turn off Heater" {
            w315 = 2.5 ("Mask")
            w323 = Kxx_Kxy_state_machine_cases."Assign Heater Current"  # States
            # "FIGURE OUT NEW HEATER CURRENT"
            n133 = Unbundle By Name(w319) -> ("Seebeck Voltage Array"=w322:dbl[], "T_H Array"=w320:dbl[], "T_C Array"=w321:dbl[], "error out"=w311:errorcluster)
            n134 = local read "Calibration Only?"() -> (w325:bool)
            n135 = local write "Mask"(w315) -> ()
            n136 = case shown="False" w325 {
              tunnel: w324 -> [w336 _]
              tunnel: w311 -> [w335 w344]
              tunnel: w320 -> [w330 _]
              tunnel: w322 -> [w331 _]
              tunnel: [w328 0.0] -> w312
              tunnel: [w337 0.0] -> w314
              tunnel: [w334 w344] -> _
              tunnel: w321 -> [w329 _]
              tunnel: [w332 0.0] -> w313
              tunnel: w315 -> [_ _]
              frame False {
                n137 = call-poly <vilib>:"Mean.vi"("X"=w331) -> ("mean"=w328:dbl)  [unwired: 1 out]
                n138 = VISA Write(VISA resource name=w336, write buffer="SOUT 0", error in (no error)=w335) -> (error out=w334:errorcluster)  [unwired: 2 out]
                n139 = call-poly <vilib>:"Mean.vi"("X"=w329) -> ("mean"=w327:dbl)  [unwired: 1 out]
                n140 = call-poly <vilib>:"Mean.vi"("X"=w330) -> ("mean"=w326:dbl)  [unwired: 1 out]
                n141 = Subtract(x=w326, y=w327) -> (x-y=w332:dbl)
                n142 = Add(x=w326, y=w327) -> (x+y=w339:dbl)
                n143 = Divide(x=w339, y=2.0) -> (x/y=w337:dbl)
                n144 = Wait (ms)(milliseconds to wait=u32 5000) -> ()  [unwired: 1 out]
              }
              frame True {
              }
            }
            n145 = local read "Global Stop"() -> (w316:bool)
            n146 = Bundle By Name(cluster=w319, "T_avg"=w314, "dTxx"=w313, "Seebeck Voltage"=w312) -> (w318:T4)
          }
          frame "Assign Heater Current" {
            n147 = local read "Preset Heater Current Array?"() -> (w351:bool)
            n148 = Unbundle By Name(w349) -> ("dTxx"=w350:dbl)
            n149 = case shown="False" w351 {
              tunnel: w350 -> [w357 _]
              tunnel: w347 -> [_ w370]
              frame False {
                n150 = local read "DeltaT (fraction of tsp)"() -> (w352:dbl)
                n151 = local read "Tsp"() -> (w359:dbl)
                n152 = Multiply(x=w352, y=w359) -> (x*y=w358:dbl)
                n153 = Divide(x=w358, y=w357) -> (x/y=w356:dbl)
                n154 = Square Root(x=w356) -> (sqrt(x)=w355:dbl)
                n155 = Less?(x=w355, y=1.6) -> (x < y?=w353:bool)
                n156 = case shown="True" w353 {
                  tunnel: w355 -> [_ w367]
                  frame False {
                    n157 = local read "HTR_Current"() -> (w361:dbl)
                    n158 = Multiply(x=w361, y=1.3) -> (x*y=w360:dbl)
                    n159 = local write "HTR_Current"(w360) -> ()
                  }
                  frame True {
                    n160 = local read "HTR_Current"() -> (w366:dbl)
                    n161 = Multiply(x=w366, y=w367) -> (x*y=w364:dbl)
                    n162 = Less?(x=w364, y=0.00075) -> (x < y?=w363:bool)
                    n163 = case shown="True" w363 {
                      tunnel: w364 -> [_ w369]
                      frame False {
                        n164 = local write "HTR_Current"(0.00075 ("HTR_Current")) -> ()
                      }
                      frame True {
                        n165 = local write "HTR_Current"(w369) -> ()
                      }
                    }
                  }
                }
              }
              frame True {
                n166 = local write "HTR_Current"(w370) -> ()
              }
            }
            n167 = local read "Global Stop"() -> (w346:bool)
          }
          frame "Plot" {
            w384 = Kxx_Kxy_state_machine_cases."End"  # States
            n168 = Unbundle By Name(w383) -> ("T_avg"=w377:dbl, "Seebeck Voltage"=w374:dbl, "dTxx"=w373:dbl)
            n169 = Divide(x=w374, y=w373) -> (x/y=w372:dbl)
            n170 = Unbundle By Name(w380) -> ("T_avg data"=w382:dbl[], "Seebeck coeff data"=w381:dbl[])
            n171 = Negate(x=w372) -> (-x=w371:dbl)
            n172 = Build Array (concatenate)(w381, w371) -> (w375:dbl[])
            n173 = Build Array (concatenate)(w382, w377) -> (w376:dbl[])
            n174 = local read "Calibration Only?"() -> (w385:bool)
            n175 = Bundle By Name(cluster=w380, "T_avg data"=w376, "Seebeck coeff data"=w375) -> (w379:T3)
            n176 = Bundle(w376, w375) -> (w386:cluster{dbl[], dbl[]})  [unwired: 1 in]
            n177 = case shown="False" w385 {
              tunnel: w386 -> [_ w387]
              frame True {
              }
              frame False {
                "Seebeck Coeff Plot" <- w387
              }
            }
            n178 = local read "Global Stop"() -> (w378:bool)
          }
          frame "End" {
          }
        }
        n179 = Wait (ms)(milliseconds to wait=u32 10) -> ()  [unwired: 1 out]
      }
      n180 = local read "Global Stop"() -> (w116:bool)
    }
    n181 = local read "Global Stop"() -> (w87:bool)
    "Fieldsp" <- w106
  }
  n182 = Less?(x="Initial Heater Current (A)", y=0.0004) -> (x < y?=w18:bool)
  n183 = case shown="True" w18 {
    tunnel: "Initial Heater Current (A)" -> [_ w393]
    frame False {
      n184 = local write "HTR_Current"(0.0004 ("HTR_Current")) -> ()
    }
    frame True {
      n185 = local write "HTR_Current"(w393) -> ()
    }
  }
  n186 = property on="Name" class="Ring (strict)"("Strings []"=w5) -> ()  [unwired: 2 in, 2 out]
  n187 = Tick Count (ms)() -> (millisecond timer value=w23:u32)
  n188 = case shown="True" "Quick Data Recording" {
    tunnel: w22 -> [_ w397]
    tunnel: "Delay (ms)" -> [_ w395]
    tunnel: w5 -> [_ w394]
    frame False {
    }
    frame True {
      # "SAVE DATA TO FILE"
      n189 = Strip Path(path=w397) -> (stripped path=w401:path, name=w398:string)
      n190 = Concatenate Strings(w398, ".dat") -> (w400:string)
      n191 = Tick Count (ms)() -> (millisecond timer value=w404:u32)
      n192 = Build Path(base path=w401, name or relative path=w400) -> (appended path=w402:path)
      n193 = call-poly <vilib>:"Write To Spreadsheet File.vi"("append to file? (new file:F)"=TRUE, "1D data"=w394, "file path (dialog if empty)"=w402) -> ("new file path (Not A Path if cancelled)"=w396:path)  [unwired: 5 in]
      n194 = while {
        tunnel: w404 -> [w429]
        tunnel: w396 -> [w421]
        tunnel: w395 -> [w420]
        stop <- w406 stop-if-true
        n195 = Wait (ms)(milliseconds to wait=w420) -> ()  [unwired: 1 out]
        n196 = Tick Count (ms)() -> (millisecond timer value=w428:u32)
        n197 = global read "MQM Data Transfer All.vi" "ZI MFLI"() -> (w408:T5)
        n198 = Subtract(x=w428, y=w429) -> (x-y=w427:u32)
        n199 = Unbundle By Name(w408) -> ("Lockin 2 Demod 0.X(V)"=w416:dbl, "Lockin 2 Demod 0.Theta (deg)"=w415:dbl)
        n200 = Unbundle By Name(w408) -> ("Lockin 3 Demod 0.X(V)"=w414:dbl, "Lockin 3 Demod 0.Theta (deg)"=w413:dbl)
        n201 = Unbundle By Name(w408) -> ("Lockin 1 Demod 0.X(V)"=w418:dbl, "Lockin 1 Demod 0.Theta (deg)"=w417:dbl)
        n202 = global read "MQM Data Transfer All.vi" "PPMS"() -> (w407:T6)
        n203 = global read "KE2182 Voltage.vi" "KE2182 Voltage (V)"() -> (w405:dbl)
        n204 = Unbundle By Name(w407) -> ("Temperature.Temperature (K)"=w426:dbl, "Field.Field (T)"=w425:dbl)
        n205 = local read "HTR_Current"() -> (w412:dbl)
        n206 = local read "I_therm"() -> (w409:dbl)
        n207 = local read "Mask"() -> (w411:dbl)
        n208 = local read "Tsp"() -> (w410:dbl)
        n209 = Build Array(w427, w426, w425, w418, w417, w416, w415, w414, w413, w405, w412, w411, w410, w409) -> (w424:dbl[])
        n210 = call "Write To Spreadsheet File (DBL)2.vi"("format (%.3f)"="%_8f", "append to file? (new file:F)"=TRUE, "1D data"=w424, "file path (dialog if empty)"=w421) -> ("error out"=w419:errorcluster)  [unwired: 3 in, 1 out]
        n211 = local read "Global Stop"() -> (w406:bool)
        n212 = call <vilib>:"Clear Errors.vi"("error in (no error)"=w419) -> ()  [unwired: 5 in, 2 out]
      }
    }
  }
  n213 = while {
    tunnel: w23 -> [w467]
    shift-right: [w461] -> _
    shift-left: 0 -> [w466]
    tunnel: w5 -> [w462]
    shift-right: [w457] -> _
    shift-left: dbl[][] [] ("array w/ subset deleted") -> [w458]
    tunnel: "Delay (ms)" -> [w451]
    stop <- "Finish" stop-if-true
    # "PLOT DATA BEING RECORDED TO FILE CONTINUOUSLY"
    n214 = Wait (ms)(milliseconds to wait=w451) -> ()  [unwired: 1 out]
    n215 = Tick Count (ms)() -> (millisecond timer value=w468:u32)
    n216 = global read "MQM Data Transfer All.vi" "ZI MFLI"() -> (w437:T5)
    n217 = Subtract(x=w468, y=w467) -> (x-y=w461:u32)
    n218 = global read "MQM Data Transfer All.vi" "PPMS"() -> (w436:T6)
    n219 = Subtract(x=w461, y=w466) -> (x-y=→"Data Rate (ms)":u32)
    n220 = Unbundle By Name(w437) -> ("Lockin 3 Demod 0.X(V)"=w440:dbl, "Lockin 3 Demod 0.Theta (deg)"=w439:dbl)
    n221 = Unbundle By Name(w437) -> ("Lockin 2 Demod 0.X(V)"=w445:dbl, "Lockin 2 Demod 0.Theta (deg)"=w454:dbl)
    n222 = Unbundle By Name(w436) -> ("Temperature.Temperature (K)"=w460:dbl, "Field.Field (T)"=w459:dbl)
    n223 = Unbundle By Name(w437) -> ("Lockin 1 Demod 0.X(V)"=w443:dbl, "Lockin 1 Demod 0.Theta (deg)"=w442:dbl)
    n224 = Build Array(w461, w460, w459) -> (w455:dbl[])
    n225 = global read "Thermometers.vi" "Thermometers"() -> (w434:cluster{"T_H":dbl, "T_C1":dbl, "T_C2":dbl})
    "Thermometers" <- w434
    n226 = Build Array (concatenate)(w455, w443, w442) -> (w453:dbl[])
    n227 = global read "KE2182 Voltage.vi" "KE2182 Voltage (V)"() -> (w430:dbl)
    "Seebeck Voltage" <- w430
    n228 = local read "HTR_Current"() -> (w450:dbl)
    n229 = Build Array (concatenate)(w453, w445, w454) -> (w441:dbl[])
    n230 = local read "I_therm"() -> (w444:dbl)
    n231 = Unbundle By Name(w434) -> ("T_H"=w433:dbl, "T_C1"=w432:dbl, "T_C2"=w431:dbl)
    n232 = Build Array (concatenate)(w441, w440, w439) -> (w438:dbl[])
    n233 = local read "Mask"() -> (w448:dbl)
    n234 = local read "Fieldsp"() -> (w435:dbl)
    n235 = local read "Tsp"() -> (w447:dbl)
    n236 = Build Array (concatenate)(w438, w430, w450, w448, w447, w444, w433, w432, w431, w435) -> (w449:dbl[])
    n237 = Build Array (concatenate)(w458, w449) -> (w452:dbl[][])
    n238 = flat-sequence {
      tunnel: "Display Elements" -> [w481]
      tunnel: [w474] -> w465
      tunnel: w462 -> [w470]
      tunnel: w452 -> [w469]
      tunnel: w465 -> [w528]
      frame #0 {
        n239 = for {
          tunnel: w481 -> [w510] mode=indexing
          shift-right: [w502] -> w480
          shift-left: dbl[] [] -> [w501]
          shift-right: [w503] -> w478
          shift-left: dbl[][] [] -> [w512]
          shift-right: [w508] -> w474
          shift-left: string[] [] -> [w507]
          tunnel: w470 -> [w504]
          tunnel: w469 -> [w505]
          i -> [w506]
          n240 = Unbundle By Name(w510) -> ("X"=w511:bool, "Y"=w514:bool, "Name"=w509:u16)
          n241 = Index Array(array=w505, index (col)=w509) -> (element=w513:dbl[])  [unwired: 1 in]
          n242 = case shown="False" w514 {
            tunnel: w513 -> [_ w520]
            tunnel: w512 -> [w518 w527]
            tunnel: [w518 w526] -> w503
            tunnel: w509 -> [_ w525]
            tunnel: [w519 w523] -> w508
            tunnel: w507 -> [w519 w522]
            tunnel: w504 -> [_ w521]
            frame False {
            }
            frame True {
              n243 = Build Array (concatenate)(w527, w520) -> (w526:dbl[][])
              n244 = Index Array(array=w521, index=w525) -> (element=w524:string)
              n245 = Build Array (concatenate)(w522, w524) -> (w523:string[])
            }
          }
          n246 = case shown="False" w511 {
            tunnel: w509 -> [_ w517]
            tunnel: w506 -> [_ _]
            tunnel: w504 -> [_ w515]
            frame False {
            }
            frame True {
              n247 = Index Array(array=w515, index=w517) -> (element=w516:string)
              n248 = property on="All Data" class="XYGraph (strict)"("XScale.NameLbl.Text"=w516) -> ()  [unwired: 2 in, 2 out]
            }
          }
          n249 = Select(t=w513, s=w511, f=w501) -> (s? t:f=w502:dbl[])
        }
        n250 = for {
          tunnel: w478 -> [w485] mode=indexing
          tunnel: w480 -> [w487]
          tunnel: [w488] -> w479 mode=indexing
          n251 = case shown="0, Default" "Y-Axis" {
            tunnel: w485 -> [w489 w491 w494]
            tunnel: [w489 w490 w493] -> w482
            frame 0, Default {
            }
            frame 1 {
              n252 = Reciprocal(x=w491) -> (1/x=w490:dbl[])
            }
            frame 2 {
              n253 = Absolute Value(x=w494) -> (abs(x)=w492:dbl[])
              n254 = Logarithm Base 10(1:w492) -> (0:w493:dbl[])
            }
          }
          n255 = case shown="0, Default" "X-Axis" {
            tunnel: w487 -> [w495 w497 w500]
            tunnel: [w495 w496 w499] -> w486
            frame 0, Default {
            }
            frame 1 {
              n256 = Reciprocal(x=w497) -> (1/x=w496:dbl[])
            }
            frame 2 {
              n257 = Absolute Value(x=w500) -> (abs(x)=w498:dbl[])
              n258 = Logarithm Base 10(1:w498) -> (0:w499:dbl[])
            }
          }
          n259 = Bundle(w486, w482) -> (w488:cluster{dbl[], dbl[]})  [unwired: 1 in]
        }
        "All Data" <- w479
        n260 = Array Size(array=w478) -> (size(s)=w477:i32[])
        n261 = Index Array(array=w477, index=0) -> (element=w475:i32)
        n262 = property on="All Data" class="XYGraph (strict)"("LegNumRows"=w475) -> ()  [unwired: 2 in, 2 out]
      }
      frame #1 {
        n263 = for {
          tunnel: w528 -> [w529] mode=indexing
          i -> [w530]
          n264 = property on="All Data" class="XYGraph (strict)"("Active Plot"=w530, "Plot.Plot Name"=w529) -> ()  [unwired: 2 in, 2 out]
        }
      }
    }
    n265 = call "Data length guard.vi"("Max length"=20000, "Array"=w452) -> ("array w/ subset deleted"=w457:dbl[][])  [unwired: 9 in]
    "Global Stop" <- "Finish"
  }
  n266 = VISA Write(VISA resource name=w3, write buffer="SOUT 0") -> (VISA resource name out=w2:refnum<visa-resource-name>)  [unwired: 1 in, 2 out]
  n267 = Unbundle By Name(w15) -> ("error out"=w14:errorcluster)
  n268 = VISA Close(VISA resource name=w11, error in (no error)=w8) -> (error out=→"KE6221 error out":errorcluster)
  n269 = VISA Close(VISA resource name=w2) -> ()  [unwired: 1 in, 1 out]
  n270 = call <instrlib>:"SetTemperature.vi"("Rate"=3.0, "Temperature"="Final Temperature (K)", "error in (no error)"=w14, "Instrument Ref In"=w12) -> ("error out"=w28:errorcluster, "Instrument Ref Out"=w29:refnum<k24>)  [unwired: 3 in, 1 out]
  n271 = call <instrlib>:"SetField.vi"("Rate"=100.0, "Field"="Final Field (Oe)", "error in (no error)"=w28, "Instrument Ref In"=w29) -> ("error out"=→"QD error out":errorcluster)  [unwired: 3 in, 2 out]
